vi "Configure Display Channels.vi"(7 "Error In":errorcluster, 9 "Channels":u8[](array[numeric]), 10 "LINX Resource":T1) -> (0 "Error Out":errorcluster, 2 "Response":u8[](array[numeric]), 3 "LINX Resource":T1)   [LabVIEW 2014, in "LMH-LINX.lvlib" / "Interaction Parts Kit.lvlib"]
doc: "Updates the Channels used in the Periodic Task using a Custom Command"
uses:
  Interaction Parts Kit.lvlib
  Private/Type Defs/LINX Ref.ctl
  Private/Type Defs/Platform.ctl
  Private/Type Defs/Interface.ctl
  Private/Device/Type Defs/LINX Device Config.ctl
  Private/Device/Type Defs/TCP Config.ctl
  Private/Device/Type Defs/Channels.ctl
  LMH-LINX.lvlib
  Private/Device/Device.lvlib
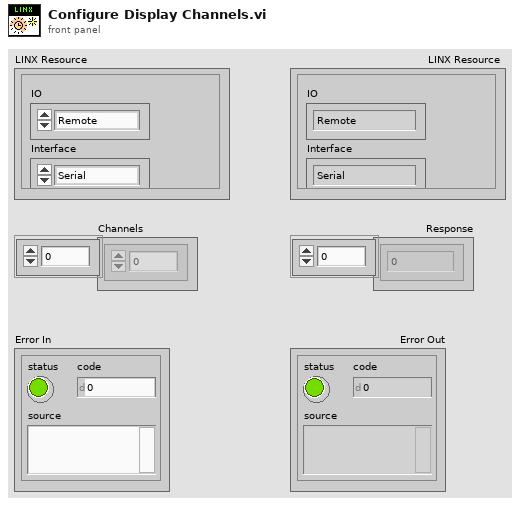
[diagram p1: front panel]
types:
  T1 = typedef "LMH-LINX.lvlib/LINX Ref.ctl" = cluster{"IO":T2, "Interface":T3, "LINX Device Config":T4}
  T2 = typedef "LMH-LINX.lvlib/Platform.ctl" = enum16{"Remote", "Local"}
  T3 = typedef "LMH-LINX.lvlib/Interface.ctl" = enum16{"Serial", "TCP"}
  T4 = typedef "LMH-LINX.lvlib/Device.lvlib/LINX Device Config.ctl" = cluster{"Interface":T3, "COM Port":refnum<visa-resource-name>, "TCP Configuration":T5, "Device Family":u8, "Device ID":u8, "Device Name":string, "TCP Ref":refnum<k5>, "Channels":T6}
  T5 = typedef "LMH-LINX.lvlib/Device.lvlib/TCP Config.ctl" = cluster{"IP Address":string, "Port":u16}
  T6 = typedef "LMH-LINX.lvlib/Channels.ctl" = cluster{"DI":u8[], "DO":u8[], "AI":u8[], "AO":u8[], "PWM":u8[], "QE":u8[], "UART":u8[], "I2C 2":u8[], "SPI":u8[], "CAN":u8[], "Servo":u8[], "AI Ref (V)":dbl, "AI Resolution (Bits)":u8, "AO Ref (V)":dbl, "AO Resolution (Bits)":u8}
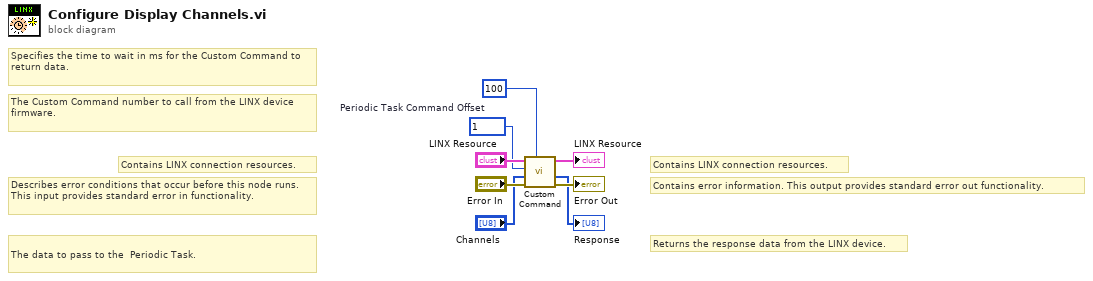
[diagram p0: block diagram]
diagram:
  w6 = u16 1  # Periodic Task Command Offset
  # "The data to pass to the  Periodic Task."
  # "Specifies the time to wait in ms for the Custom Command to return data."
  # "The Custom Command number to call from the LINX device firmware."
  # "Returns the response data from the LINX device."
  # "Contains LINX connection resources."
  # "Contains error information. This output provides standard error out functionality."
  # "Contains LINX connection resources."
  # "Describes error conditions that occur before this node runs. This input provides standard error in functionality."
  n1 = call "Custom Command.vi"("Timeout (100 ms)"=100, "Error In"="Error In", "Data"="Channels", "Custom Command Number"=w6, "LINX Resource"="LINX Resource") -> ("Error Out"=→"Error Out":errorcluster, "Response"=→"Response":u8[], "LINX Resource"=→"LINX Resource":T1)  [unwired: 3 in, 1 out]
